vi "wrap count.vi"(10 "lo":u16, 11 "hi":u16) -> (3 "Numeric":dbl)   [LabVIEW 2025, in "Motor.lvlib" / "CL57RS.lvclass"]
uses:
  Stepper/Stepper.lvclass/Stepper.ctl
  CL57RS.lvclass
  CL57RS.lvclass/CL57RS.ctl
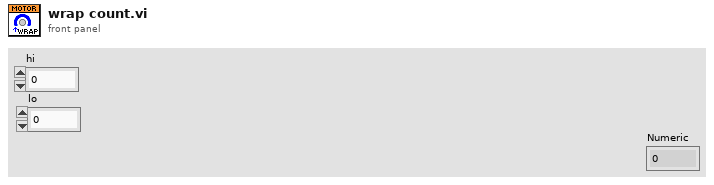
[diagram p1: front panel]
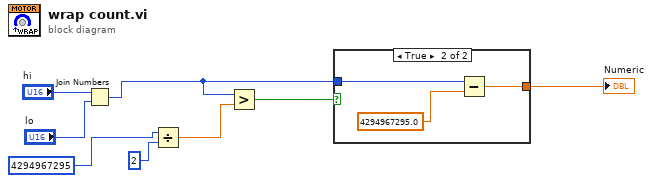
[diagram p0: block diagram]
diagram:
  n1 = Join Numbers(hi="hi", lo="lo") -> ((hi.lo)=w3:u32)
  n2 = Divide(x=u32 4294967295, y=u32 2) -> (x/y=w5:dbl)
  n3 = Greater?(x=w3, y=w5) -> (0:w4:bool)
  n4 = case shown="True" w4 {
    tunnel: w3 -> [w9 w11]
    tunnel: [w9 w10] -> w2
    frame False {
    }
    frame True {
      n5 = Subtract(x=w11, y=4294967295.0 ("(hi.lo)")) -> (x-y=w10:dbl)
    }
  }
  "Numeric" <- w2
